vi "Stepper.vi"() -> ()   [LabVIEW 2020]
uses:
  <vilib>/LabVIEW Interface for Arduino/LabVIEW Interface for Arduino.lvlib
panel:
  in  "Auto Refersh":bool
  in  "Auto OFF":bool
  in  "Steps to Move 1*":i16
  in  "Stepper Pins*":u8
  in  "Auto Start":bool
  in  "Steps to Move 1":i16
  in  "Stepper Pins":u8
  in  "Stepper Motor Control":bool
  in  "Program Stop":bool
  in  "VISA resource":refnum<visa-resource-name>
  # "Auto & Manual"
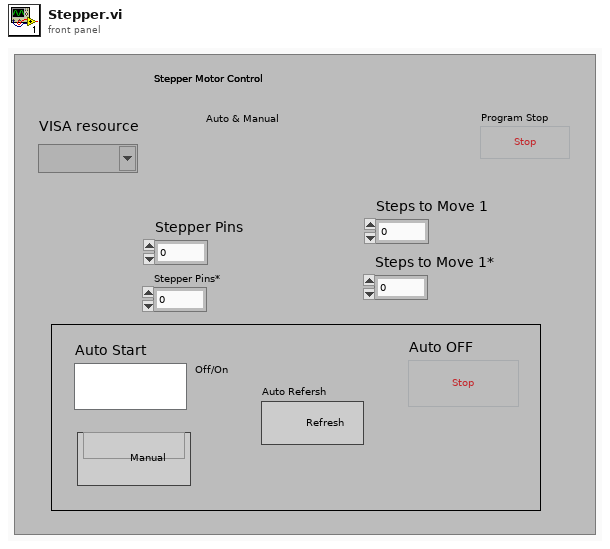
[diagram p1: front panel]
types:
  T1 = typedef "LabVIEW Interface for Arduino.lvlib/Arduino Resource.ctl" = cluster{"VISA resource":refnum<visa-resource-name>, "Board Type":T2, "Connection Type":enum8{"USB / Serial"}, "Bytes Per Packet (15)":u8}
  T2 = typedef "LabVIEW Interface for Arduino.lvlib/Board Type.ctl" = enum16{"Uno", "Dimuelanove w/Atmega 328", "Mega 2560"}
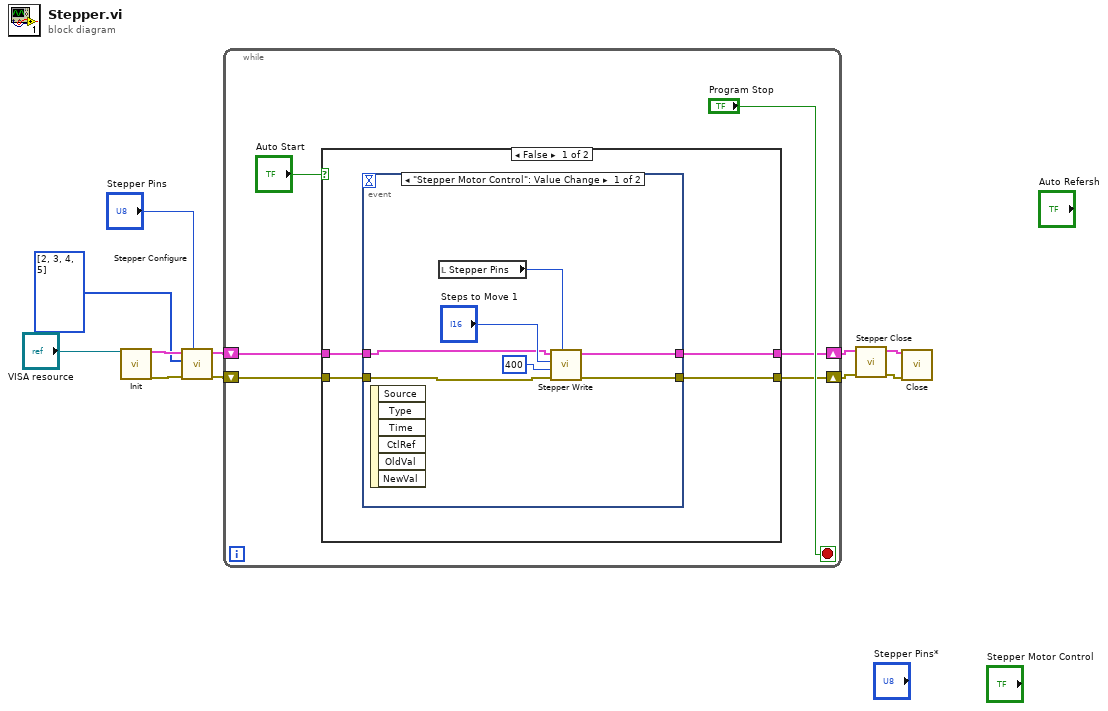
[diagram p0: block diagram]
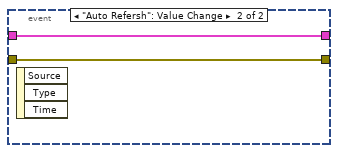
[diagram p2: hidden frame]
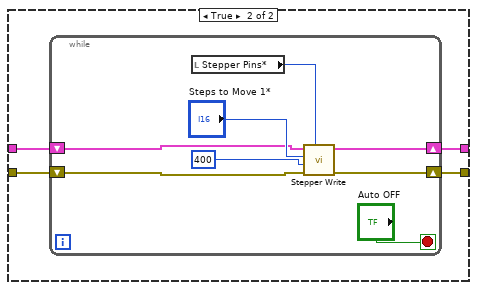
[diagram p3: hidden frame]
diagram:
  n1 = call <vilib>:"Init.vi"("VISA resource"="VISA resource") -> ("Arduino Resource"=w11:T1, "error out"=w10:errorcluster)  [unwired: 17 in]
  n2 = call <vilib>:"Stepper Configure.vi"("Stepper #"="Stepper Pins", "error in"=w10, "Stepper Pins"=u8[] [2, 3, 4, 5], "Arduino Resource"=w11) -> ("error out"=w6:errorcluster, "Arduino Resource Out"=w7:T1)  [unwired: 6 in]
  n3 = while {
    shift-right: [w13] -> w5
    shift-left: w7 -> [w15]
    shift-right: [w12] -> w4
    shift-left: w6 -> [w14]
    stop <- "Program Stop" stop-if-true
    n4 = case shown="False" "Auto Start" {
      tunnel: [w19 w34] -> w13
      tunnel: [w18 w33] -> w12
      tunnel: w15 -> [w21 w32]
      tunnel: w14 -> [w20 w31]
      frame False {
        n5 = event shown="[0] \"Stepper Motor Control\": Value Change" {
          selector: _ -> [_ _]
          dyn-events: _ -> [_ _]
          timeout: _ -> [_ _]
          tunnel: w21 -> [w23 w30]
          tunnel: [w25 w30] -> w19
          tunnel: [w24 w29] -> w18
          tunnel: w20 -> [w22 w29]
          event "Stepper Motor Control": Value Change {
            n6 = event-data() -> ()  [unwired: 1 in, 6 out]
            n7 = local read "Stepper Pins"() -> (w28:u8)
            n8 = call <vilib>:"Stepper Write.vi"("Stepper #"=w28, "error in"=w22, "Set Speed (Steps per Second)"=i16 400, "# of Steps to Move"="Steps to Move 1", "Arduino Resource"=w23) -> ("error out"=w24:errorcluster, "Arduino Resource Out"=w25:T1)  [unwired: 5 in]
          }
          event "Auto Refersh": Value Change {
            n9 = event-data() -> ()  [unwired: 1 in, 3 out]
          }
        }
      }
      frame True {
        n10 = while {
          shift-right: [w40] -> w34
          shift-left: w32 -> [w38]
          shift-right: [w39] -> w33
          shift-left: w31 -> [w37]
          stop <- "Auto OFF" stop-if-true
          n11 = local read "Stepper Pins*"() -> (w35:u8)
          n12 = call <vilib>:"Stepper Write.vi"("Stepper #"=w35, "error in"=w37, "Set Speed (Steps per Second)"=i16 400, "# of Steps to Move"="Steps to Move 1*", "Arduino Resource"=w38) -> ("error out"=w39:errorcluster, "Arduino Resource Out"=w40:T1)  [unwired: 5 in]
        }
      }
    }
  }
  n13 = call <vilib>:"Stepper Close.vi"("error in"=w4, "Arduino Resource"=w5) -> ("error out"=w2:errorcluster, "Arduino Resource Out"=w3:T1)  [unwired: 8 in]
  n14 = call <vilib>:"Close.vi"("Arduino Resource"=w3, "error in"=w2) -> ()  [unwired: 13 in, 1 out]
